vi "Write Channel Name.vi"(8 "error in":errorcluster, 10 "channel name":string, 11 "cRIO repo in":refnum<class "cRIORepo.lvclass">) -> (0 "error out":errorcluster, 3 "cRIO repo out":refnum<class "cRIORepo.lvclass">)   [LabVIEW 2015, in "cRIORepo.lvclass"]
uses:
  cRIORepo.lvclass
  cRIORepo.lvclass/cRIORepo.ctl
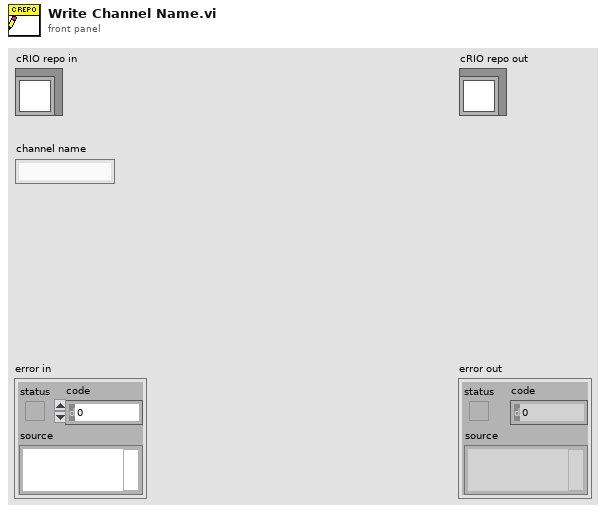
[diagram p1: front panel]
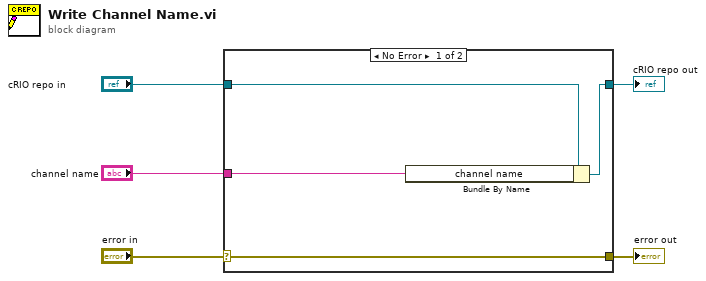
[diagram p0: block diagram]
diagram:
  n1 = case shown="No Error" "error in" {
    selector: "error in" -> [w9 w10]
    tunnel: [w9 w10] -> w4
    tunnel: [w7 w11] -> w2
    tunnel: "cRIO repo in" -> [w8 w11]
    tunnel: "channel name" -> [w6 _]
    frame No Error {
      n2 = Bundle By Name(cluster=w8, "channel name"=w6) -> (w7:refnum<class "cRIORepo.lvclass">)
    }
    frame Error {
    }
  }
  "error out" <- w4
  "cRIO repo out" <- w2
